vi "Set FIle Extension to Match.vi"(8 "error in":errorcluster, 10 "Path to Binary File to Verify":path, 11 "Options in":refnum<class "Options.lvclass">) -> (0 "error out":errorcluster, 3 "Options out":refnum<class "Options.lvclass">)   [LabVIEW 2020, in "Approval Tests.lvlib" / "Options.lvclass"]
uses:
  Options.lvclass
  Options.lvclass/Options.ctl
  Naming Data/Naming Data.lvclass/Naming Data.ctl
  Read Naming Data.vi
  Naming Data/Read Extension.vi
  Naming Data/Write Extension.vi
  Write Naming Data.vi
  Naming Data/Naming Data.lvclass
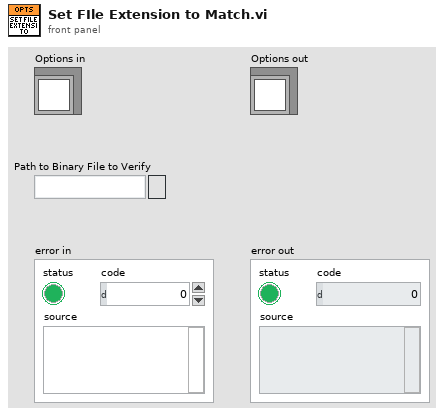
[diagram p1: front panel]
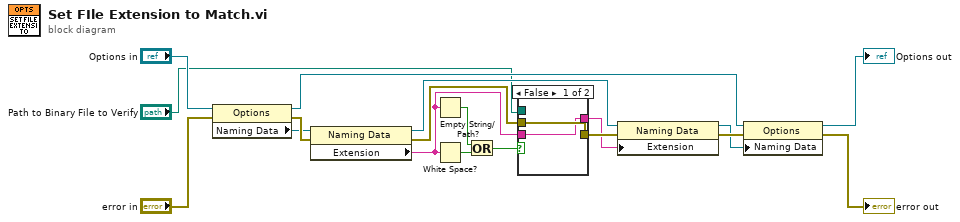
[diagram p0: block diagram]
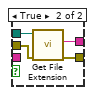
[diagram p2: hidden frame]
diagram:
  n1 = property on="Property Node" class="Options"(reference="Options in", error in="error in") -> (reference out=w9:refnum<class "Options.lvclass">, error out=w14:errorcluster, "Naming Data"=w6:refnum<class "Naming Data.lvclass">)
  n2 = property on="Property Node" class="Naming Data"(reference=w6, error in=w14) -> (reference out=w10:refnum<class "Naming Data.lvclass">, error out=w15:errorcluster, "Extension"=w11:string)
  n3 = Empty String/Path?(string/path=w11) -> (empty?=w1:bool)
  n4 = White Space?(1:w11) -> (0:w2:bool)
  n5 = Or(x=w1, y=w2) -> (x .or. y?=w3:bool)
  n6 = case shown="False" w3 {
    tunnel: "Path to Binary File to Verify" -> [_ w22]
    tunnel: [w19 w21] -> w5
    tunnel: w11 -> [w19 _]
    tunnel: w15 -> [w20 w24]
    tunnel: [w20 w23] -> w16
    frame False {
    }
    frame True {
      n7 = call <vilib>:"Get File Extension.vi"("error in (no error)"=w24, "file"=w22) -> ("error out"=w23:errorcluster, "lowercase file extension"=w21:string)  [unwired: 5 in, 3 out]
    }
  }
  n8 = property on="Property Node" class="Naming Data"(reference=w10, error in=w16, "Extension"=w5) -> (reference out=w7:refnum<class "Naming Data.lvclass">, error out=w17:errorcluster)
  n9 = property on="Property Node" class="Options"(reference=w9, error in=w17, "Naming Data"=w7) -> (reference out=→"Options out":refnum<class "Options.lvclass">, error out=→"error out":errorcluster)
